vi "GetAppInfoInClusterArray.vi"(0 "Array":cluster{"App Refnum":refnum<vi>}[](array[cluster])) -> (1 "VI Version":string, 2 "Application:User Name":string, 3 "Operating System:Name":string, 4 "error out":errorcluster)   [LabVIEW 2013]
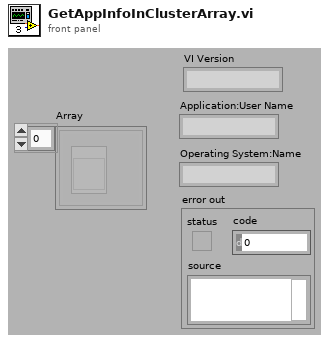
[diagram p1: front panel]
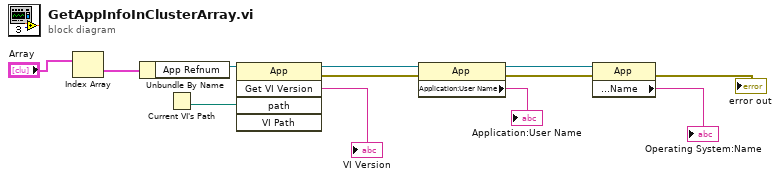
[diagram p0: block diagram]
diagram:
  n1 = Index Array(array="Array") -> (element=w1:cluster{"App Refnum":refnum<vi>})  [unwired: 1 in]
  n2 = Unbundle By Name(w1) -> ("App Refnum"=w2:refnum<vi>)
  n3 = Current VI's Path() -> (path=w12:path)
  n4 = invoke class="App" method="Get VI Version"(reference=w2, "path"=w12) -> (reference out=w10:refnum<vi>, error out=w9:errorcluster, "GetVIVers"=→"VI Version":string)  [unwired: 3 in, 2 out]
  n5 = property class="App"(reference=w10, error in=w9) -> (reference out=w8:refnum<vi>, error out=w7:errorcluster, "Application:User Name"=→"Application:User Name":string)
  n6 = property class="App"(reference=w8, error in=w7) -> (error out=→"error out":errorcluster, "Operating System:Name"=→"Operating System:Name":string)  [unwired: 1 out]
